vi "tt20panel_update_counts.vi"(8 "error in (no error)":errorcluster, 10 "Counts":dbl[](array[numeric]), 11 "tt20panel in":refnum<class "tt20panel.lvclass">) -> (0 "error out":errorcluster, 3 "tt20panel out":refnum<class "tt20panel.lvclass">)   [LabVIEW 2015, in "tt20panel.lvclass"]
uses:
  tt20panel.lvclass
  UI/panel_class/panel.lvclass/panel.ctl
  tt20panel.lvclass/tt20panel.ctl
  UI/panel_class/panel.lvclass
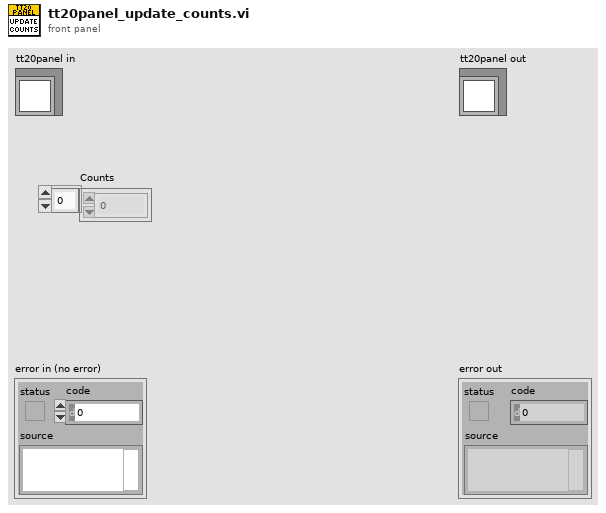
[diagram p1: front panel]
types:
  T1 = typedef "ui_user_events.ctl" = cluster{"update_xy_graph":refnum<user-event>, "update_graph":refnum<user-event>, "update_chart":refnum<user-event>, "update_map":refnum<user-event>, "event_loop_stop":refnum<user-event>, "keep_map":refnum<user-event>}
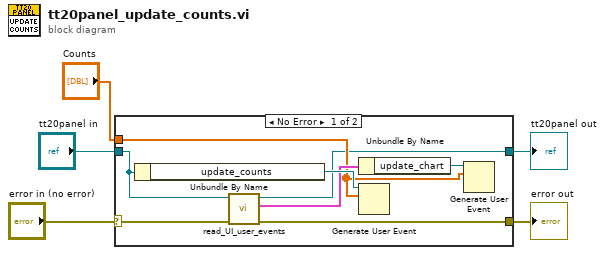
[diagram p0: block diagram]
diagram:
  n1 = case shown="No Error" "error in (no error)" {
    selector: "error in (no error)" -> [w11 w15]
    tunnel: [w6 w15] -> w4
    tunnel: [w7 w14] -> w2
    tunnel: "tt20panel in" -> [w12 w14]
    tunnel: "Counts" -> [w8 _]
    frame No Error {
      n2 = Unbundle By Name(w12) -> ("update_counts"=w13:refnum<user-event>)
      n3 = call "read_UI_user_events.vi"("error in (no error)"=w11, "panel in"=w12) -> ("error out"=w6:errorcluster, "ui_user_events"=w10:T1, "panel out"=w7:refnum<class "tt20panel.lvclass">)  [unwired: 7 in]
      n4 = Unbundle By Name(w10) -> ("update_chart"=w9:refnum<user-event>)
      n5 = Generate User Event(user event=w13, event data cluster=w8) -> ()  [unwired: 2 in, 2 out]
      n6 = Generate User Event(user event=w9, event data cluster=w8) -> ()  [unwired: 2 in, 2 out]
    }
    frame Error {
    }
  }
  "error out" <- w4
  "tt20panel out" <- w2
